vi "VLC - Convert Video to mp4-1.vi"(5 "Path":path, 11 "error in (no error)":errorcluster) -> (15 "error out":errorcluster)   [LabVIEW 2009]
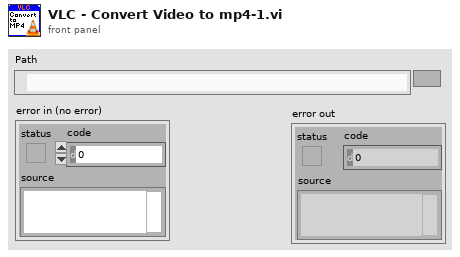
[diagram p1: front panel]
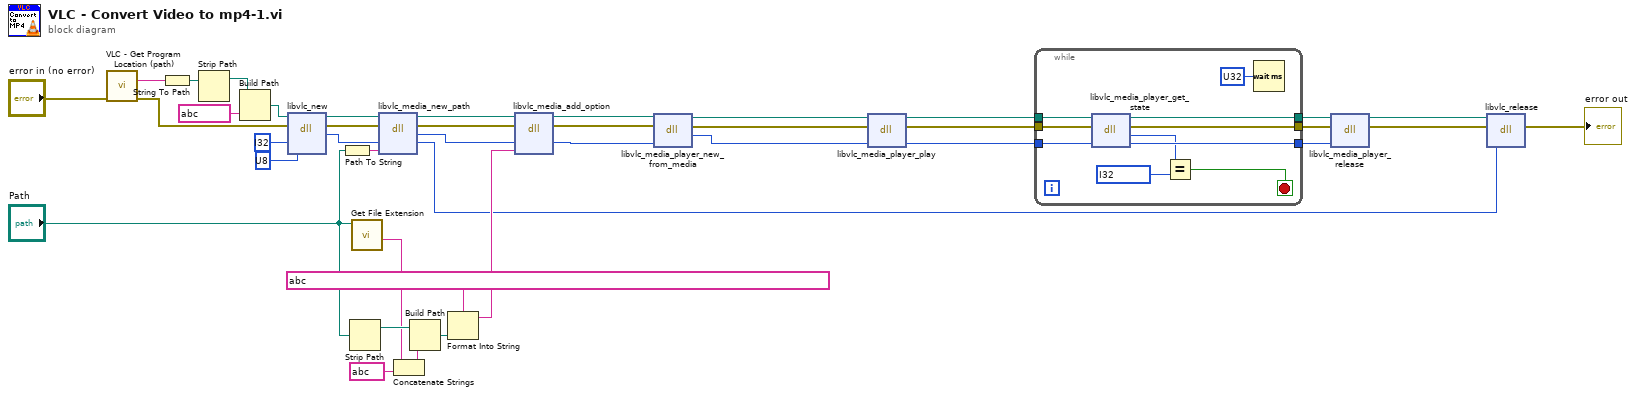
[diagram p0: block diagram]
diagram:
  n1 = call "VLC - Get Program Location (path).vi"("error in (no error)"="error in (no error)") -> ("VLC path"=w34:string, "error out"=w9:errorcluster)  [unwired: 13 in]
  n2 = String To Path(string=w34) -> (path=w38:path)
  n3 = Strip Path(path=w38) -> (stripped path=w37:path)  [unwired: 1 out]
  n4 = Build Path(base path=w37, name or relative path=string ?) -> (appended path=w35:path)
  n5 = dll-call lib="C:/Program Files (x86)/VideoLAN/VLC/libvlc.dll" fn="libvlc_new"(path in=w35, error in=w9, "argc"=i32 ?, "argv"=u8 ?) -> (path out=w33:path, error out=w32:errorcluster, "return type"=w31:i32)  [unwired: 3 in]
  n6 = Path To String(path="Path") -> (string=w30:string)
  n7 = Strip Path(path="Path") -> (stripped path=w23:path)  [unwired: 1 out]
  n8 = call <vilib>:"Get File Extension.vi"("file"="Path") -> ("filename without extension"=w21:string)  [unwired: 6 in, 4 out]
  n9 = dll-call lib="C:/Program Files (x86)/VideoLAN/VLC/libvlc.dll" fn="libvlc_media_new_path"(path in=w33, error in=w32, "p_instance"=w31, "path"=w30) -> (path out=w29:path, error out=w28:errorcluster, "return type"=w27:i32, "p_instance"=w11:i32)  [unwired: 2 in]
  n10 = Concatenate Strings(w21, string ? ("string")) -> (w20:string)
  n11 = Build Path(base path=w23, name or relative path=w20) -> (appended path=w22:path)
  n12 = Format Into String(format string=string ?, w22) -> (resulting string=w25:string)  [unwired: 2 in, 1 out]
  n13 = dll-call lib="C:/Program Files (x86)/VideoLAN/VLC/libvlc.dll" fn="libvlc_media_add_option"(path in=w29, error in=w28, "p_md"=w27, "ppsz_options"=w25) -> (path out=w18:path, error out=w17:errorcluster, "p_md"=w7:i32)  [unwired: 3 in]
  n14 = dll-call lib="C:/Program Files (x86)/VideoLAN/VLC/libvlc.dll" fn="libvlc_media_player_new_from_media"(path in=w18, error in=w17, "p_md"=w7) -> (path out=w16:path, error out=w15:errorcluster, "return type"=w14:i32)  [unwired: 2 in]
  n15 = dll-call lib="C:/Program Files (x86)/VideoLAN/VLC/libvlc.dll" fn="libvlc_media_player_play"(path in=w16, error in=w15, "p_mi"=w14) -> (path out=w6:path, error out=w5:errorcluster, "p_mi"=w4:i32)  [unwired: 2 in]
  n16 = while {
    tunnel: w6 -> [w50]
    tunnel: w5 -> [w49]
    tunnel: w4 -> [w48]
    tunnel: [w47] -> w3
    tunnel: [w46] -> w2
    tunnel: [w45] -> w1
    stop <- w42 stop-if-true
    w43 = i32 ? items=["IDLE/CLOSE", "OPENING", "BUFFERING", "PLAYING", "PAUSED", "STOPPING", "ENDED", "ERROR"] ("Ring")
    n17 = dll-call lib="C:/Program Files (x86)/VideoLAN/VLC/libvlc.dll" fn="libvlc_media_player_get_state"(path in=w50, error in=w49, "p_mi"=w48) -> (path out=w46:path, error out=w45:errorcluster, "return type"=w44:i32, "p_mi"=w47:i32)  [unwired: 1 in]
    n18 = Equal?(x=w44, y=w43) -> (x = y?=w42:bool)
    n19 = Wait (ms)(milliseconds to wait=u32 ?) -> ()  [unwired: 1 out]
  }
  n20 = dll-call lib="C:/Program Files (x86)/VideoLAN/VLC/libvlc.dll" fn="libvlc_media_player_release"(path in=w2, error in=w1, "p_mi"=w3) -> (path out=w13:path, error out=w12:errorcluster)  [unwired: 3 in]
  n21 = dll-call lib="C:/Program Files (x86)/VideoLAN/VLC/libvlc.dll" fn="libvlc_release"(path in=w13, error in=w12, "p_instnace"=w11) -> (error out=→"error out":errorcluster)  [unwired: 3 in, 1 out]
